vi "Write TC Temperature.vi"(8 "error in (no error)":errorcluster, 10 "TC Temperature":waveform(dbl)[](array[waveform]), 11 "Results in":refnum<class "Cryo Sep Results.lvclass">) -> (0 "error out":errorcluster, 3 "Results out":refnum<class "Cryo Sep Results.lvclass">)   [LabVIEW 2019, in "Results.lvlib" / "Cryo Sep Results.lvclass"]
uses:
  Cryo Sep Results.lvclass
  Cryo Sep Results.lvclass/Cryo Sep Results.ctl
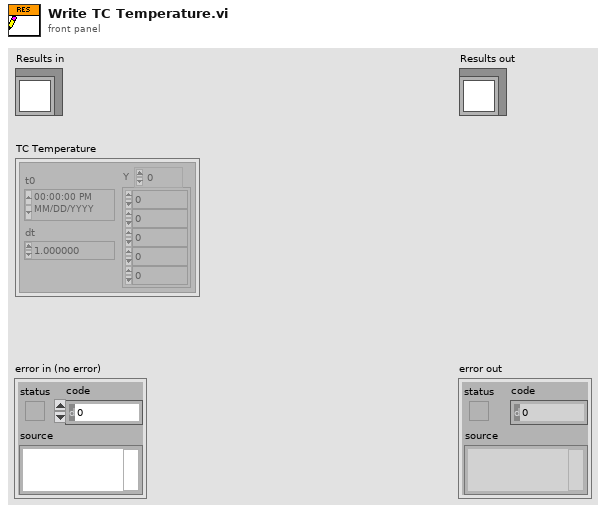
[diagram p1: front panel]
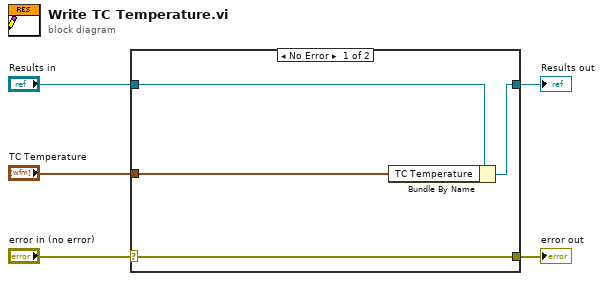
[diagram p0: block diagram]
diagram:
  n1 = case shown="No Error" "error in (no error)" {
    selector: "error in (no error)" -> [w9 w10]
    tunnel: [w9 w10] -> w4
    tunnel: [w7 w11] -> w2
    tunnel: "Results in" -> [w8 w11]
    tunnel: "TC Temperature" -> [w6 _]
    frame No Error {
      n2 = Bundle By Name(cluster=w8, "TC Temperature"=w6) -> (w7:refnum<class "Cryo Sep Results.lvclass">)
    }
    frame Error {
    }
  }
  "error out" <- w4
  "Results out" <- w2
